vi "MeasureBaselineCurrents.vi"   [LabVIEW 2023]
doc: "Measures and reports the baseline PDH currents during a systems check."
uses:
  GlobalDriverStationData.vi
  GlobalAutonomous.vi
  GlobalMiscellaneous.vi
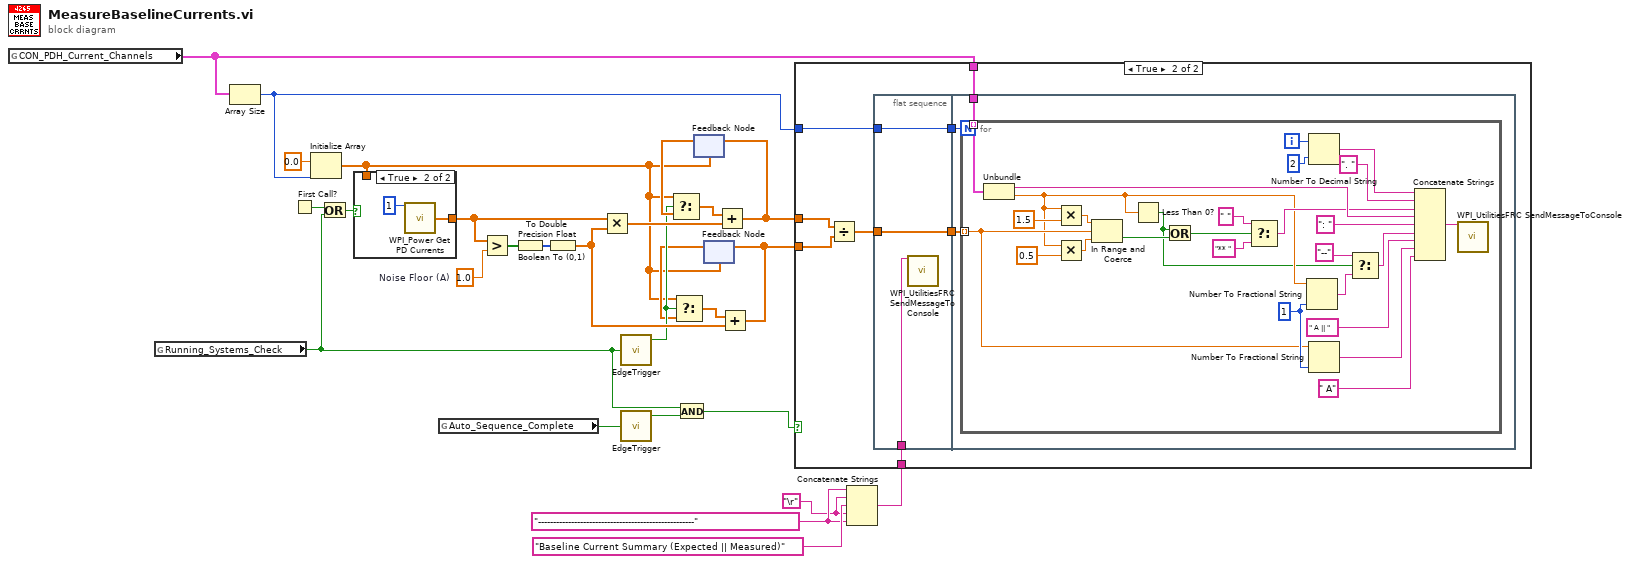
[diagram p0: block diagram]
diagram:
  w7 = "----------------------------------------------------" ("string")
  w6 = "\r"
  w24 = 1.0  # Noise Floor (A)
  n1 = global read "GlobalMiscellaneous.vi" "CON_PDH_Current_Channels"() -> (w1:cluster{string, dbl}[])
  n2 = global read "GlobalDriverStationData.vi" "Running_Systems_Check"() -> (w4:bool)
  n3 = Array Size(array=w1) -> (size(s)=w8:i32)
  n4 = First Call?() -> (First Call?: T/F=w12:bool)
  n5 = Initialize Array(0.0 ("element"), w8) -> (w11:dbl[])
  n6 = Or(x=w12, y=w4) -> (x .or. y?=w13:bool)
  n7 = case shown="True" w13 {
    tunnel: [w28 w29] -> w21
    tunnel: w11 -> [w28 _]
    frame False {
    }
    frame True {
      n8 = call <vilib>:"WPI_Power Get PD Currents.vi"("Power Distribution (def)"=u8 1) -> ("all currents (A)"=w29:dbl[])  [unwired: 11 in, 3 out]
    }
  }
  n9 = global read "GlobalAutonomous.vi" "Auto_Sequence_Complete"() -> (w5:bool)
  n10 = Greater?(x=w21, y=w24) -> (0:w23:bool[])
  n11 = Boolean To (0,1)(Boolean=w23) -> (0, 1=w22:i16[])
  n12 = To Double Precision Float(number=w22) -> (double precision float=w18:dbl[])
  n13 = Multiply(x=w21, y=w18) -> (x*y=w20:dbl[])
  n14 = call "EdgeTrigger.vi"("Input Signal"=w4) -> ("Rising Edge Trigger"=w17:bool)  [unwired: 2 out]
  n15 = call "EdgeTrigger.vi"("Input Signal"=w5) -> ("Rising Edge Trigger"=w2:bool)  [unwired: 2 out]
  n16 = And(x=w4, y=w2) -> (x .and. y?=w3:bool)
  n17 = feedback #1(w11) -> (w26:dbl[])
  n18 = Select(t=w11, s=w17, f=w26) -> (s? t:f=w25:dbl[])
  n19 = feedback #2(w11) -> (w16:dbl[])
  n20 = Select(t=w11, s=w17, f=w16) -> (s? t:f=w19:dbl[])
  n21 = Add(x=w25, y=w20) -> (x+y=w15:dbl[])
  n22 = feedback-in #1(w15) -> ()
  n23 = Add(x=w19, y=w18) -> (x+y=w14:dbl[])
  n24 = feedback-in #2(w14) -> ()
  n25 = Concatenate Strings(w7, w6, "Baseline Current Summary (Expected || Measured)" ("Message"), w6, w7) -> (w10:string)
  n26 = case shown="True" w3 {
    tunnel: w15 -> [_ w38]
    tunnel: w14 -> [_ w37]
    tunnel: w8 -> [_ w35]
    tunnel: w10 -> [_ w32]
    tunnel: w1 -> [_ w31]
    frame False {
    }
    frame True {
      n27 = Divide(x=w38, y=w37) -> (x/y=w36:dbl[])
      n28 = flat-sequence {
        tunnel: w35 -> [w40]
        tunnel: w36 -> [w41]
        tunnel: [w41] -> w34
        tunnel: [w40] -> w33
        tunnel: w32 -> [w39]
        tunnel: w34 -> [w44]
        tunnel: w33 -> [w43]
        tunnel: w31 -> [w42]
        frame #0 {
          n29 = call <vilib>:"WPI_UtilitiesFRC SendMessageToConsole.vi"("Message"=w39) -> ()  [unwired: 14 in, 1 out]
        }
        frame #1 {
          n30 = for {
            N: w43 -> [_]
            tunnel: w44 -> [w53] mode=indexing
            tunnel: w42 -> [w66] mode=indexing
            i -> [w57]
            w68 = i16 1 ("precision (6)")
            n31 = Unbundle(w66) -> (w65:string, w52:dbl)
            n32 = Multiply(x=w52, y=1.5) -> (x*y=w64:dbl)
            n33 = Multiply(x=w52, y=0.5) -> (x*y=w63:dbl)
            n34 = In Range and Coerce(upper limit=w64, x=w53, lower limit=w63) -> (In Range?=w51:bool)  [unwired: 1 out]
            n35 = Less Than 0?(x=w52) -> (x < 0?=w48:bool)
            n36 = Or(x=w48, y=w51) -> (x .or. y?=w50:bool)
            n37 = Select(t=" ", s=w50, f="** ") -> (s? t:f=w60:string)
            n38 = Number To Fractional String(number=w52, precision (6)=w68) -> (F-format string=w46:string)  [unwired: 2 in]
            n39 = Number To Decimal String(number=w57, width (-)=i16 2) -> (decimal integer string=w55:string)
            n40 = Number To Fractional String(number=w53, precision (6)=w68) -> (F-format string=w47:string)  [unwired: 2 in]
            n41 = Select(t="--", s=w48, f=w46) -> (s? t:f=w45:string)
            n42 = Concatenate Strings(w55, ". " ("string"), w60, w65, ": ", w45, " A || ", w47, " A") -> (w67:string)
            n43 = call <vilib>:"WPI_UtilitiesFRC SendMessageToConsole.vi"("Message"=w67) -> ()  [unwired: 14 in, 1 out]
          }
        }
      }
    }
  }
